vi "CANXNETInit.vi"(8 "Double":bool=TRUE, 11 "BaudRate":u32=500000) -> (3 "XNET out":T1)   [LabVIEW 2017]
doc: "This example demonstrates frame streaming input using an NI-XNET Frame Input session. \n\nThis example can run against any output example, assuming you have a properly terminated CAN cable connected to two CAN ports.\n\nIf you have no database aliases on your system, the example automatically loads the nixnet_example database."
uses:
  <vilib>/xnet/xnet.llb/XNET Create Session (Frame Input Stream).vi
  <vilib>/xnet/xnet.llb/XNET Create Session (Frame Output Stream).vi
  <resource>/objmgr/xnet.rc
panel:
  in  "Echo Transmit?":bool
  in  "Termination?":u32(ring) items=["Off", "On"]
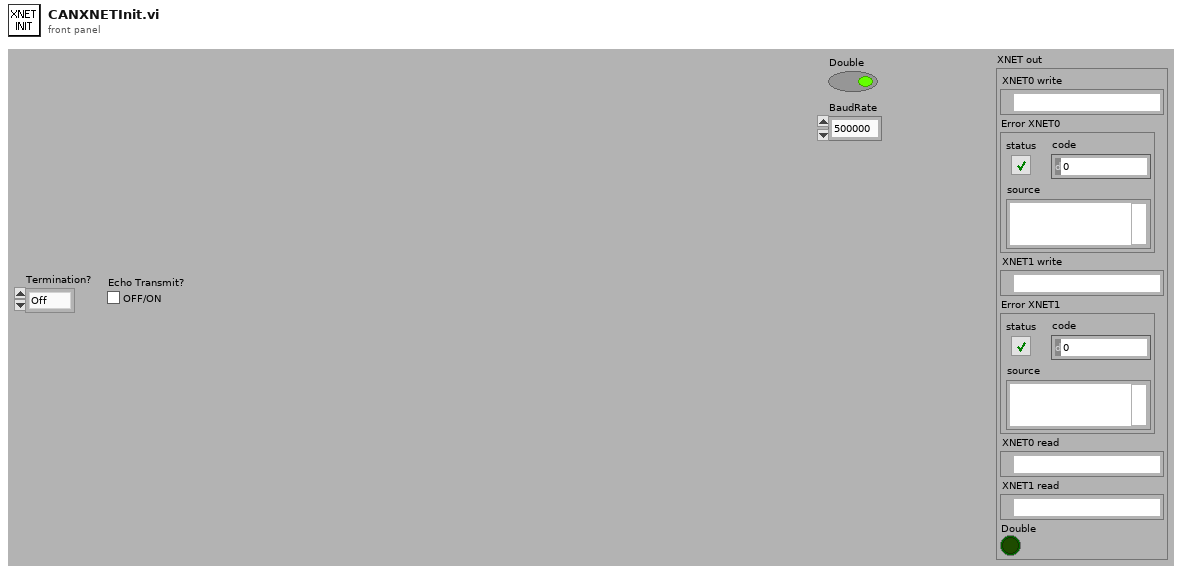
[diagram p1: front panel]
types:
  T1 = cluster{"XNET0 write":refnum<k21>, "Error XNET0":errorcluster, "XNET1 write":refnum<k21>, "Error XNET1":errorcluster, "XNET0 read":refnum<k21>, "XNET1 read":refnum<k21>, "Double":bool}
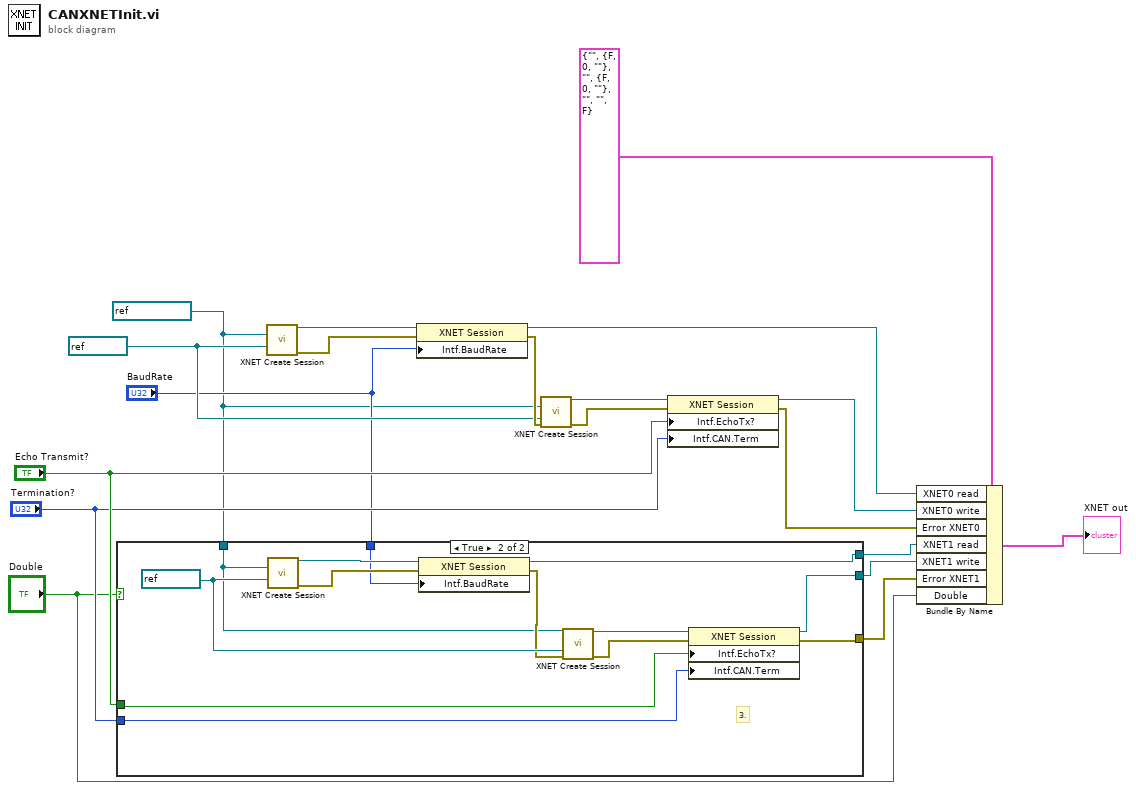
[diagram p0: block diagram]
diagram:
  w3 = refnum<k21> "CAN2" ("Select Interface")
  w1 = refnum<k21> ":memory:" ("CAN Cluster")
  n1 = case shown="True" "Double" {
    tunnel: w1 -> [_ w20]
    tunnel: "Termination?" -> [_ w28]
    tunnel: "Echo Transmit?" -> [_ w27]
    tunnel: [_ w24] -> w9
    tunnel: [_ w23] -> w8
    tunnel: [_ w22] -> w7
    tunnel: "BaudRate" -> [_ w21]
    frame False {
    }
    frame True {
      w26 = refnum<k21> "CAN3" ("Select Interface")
      # "3."
      n2 = call-poly <vilib>:"XNET Create Session.vi"("cluster (:memory:)"=w20, "interface"=w26) -> ("session out"=w31:refnum<k21>, "error out"=w32:errorcluster)  [unwired: 1 in, 11 out]
      n3 = property class="XNET Session"(reference=w31, error in=w32, "Intf.BaudRate"=w21) -> (reference out=w22:refnum<k21>, error out=w25:errorcluster)
      n4 = call-poly <vilib>:"XNET Create Session.vi"("cluster (:memory:)"=w20, "interface"=w26, "error in (no error)"=w25) -> ("session out"=w30:refnum<k21>, "error out"=w29:errorcluster)  [unwired: 11 out]
      n5 = property class="XNET Session"(reference=w30, error in=w29, "Intf.EchoTx?"=w27, "Intf.CAN.Term"=w28) -> (reference out=w23:refnum<k21>, error out=w24:errorcluster)
    }
  }
  n6 = call-poly <vilib>:"XNET Create Session.vi"("cluster (:memory:)"=w1, "interface"=w3) -> ("session out"=w19:refnum<k21>, "error out"=w18:errorcluster)  [unwired: 1 in, 11 out]
  n7 = property class="XNET Session"(reference=w19, error in=w18, "Intf.BaudRate"="BaudRate") -> (reference out=w15:refnum<k21>, error out=w6:errorcluster)
  n8 = call-poly <vilib>:"XNET Create Session.vi"("cluster (:memory:)"=w1, "interface"=w3, "error in (no error)"=w6) -> ("session out"=w14:refnum<k21>, "error out"=w13:errorcluster)  [unwired: 11 out]
  n9 = property class="XNET Session"(reference=w14, error in=w13, "Intf.EchoTx?"="Echo Transmit?", "Intf.CAN.Term"="Termination?") -> (reference out=w5:refnum<k21>, error out=w4:errorcluster)
  n10 = Bundle By Name(cluster=T1 {"XNET0 write"="", "Error XNET0"={"status"=FALSE, "code"=0, "source"=""}, "XNET1 write"="", "Error XNET1"={"status"=FALSE, "code"=0, "source"=""}, "XNET0 read"="", "XNET1 read"="", "Double"=FALSE} ("XNET out"), "XNET0 read"=w15, "XNET0 write"=w5, "Error XNET0"=w4, "XNET1 read"=w7, "XNET1 write"=w8, "Error XNET1"=w9, "Double"="Double") -> (→"XNET out":T1)
